vi "Teleop.vi"(10 "Match Info":T1={"Autonomous Elapsed Seconds"=0.0, "TeleOp Elapsed Seconds"=0.0, "Disabled Elapsed Seconds"=0.0, "Visited Autonomous"=FALSE, "Visited TeleOp"=FALSE, "Visited Disabled"=FALSE, "Autonomous Settings"={"Autonomous Style"=enum."Independent", "VI Refnum"=refnum}}, 11 "Call Context":T2) -> ()   [LabVIEW 2017]
doc: "This VI is called for each TeleOp packet received from the DS where the robot is not disabled. It is often used to read from the joysticks and update I/O or to update setpoints for timed control loops. It should complete and return within 20 milliseconds or it may miss DS packets."
uses:
  <vilib>/Rock Robotics/WPI/DriverStation/WPI_DriverStationDerivedRobotMode.ctl
  <vilib>/Rock Robotics/WPI/DriverStation/WPI_DriverStationMatch Info.ctl
  <vilib>/Rock Robotics/WPI/Utilities/WPI_GetSetVariantRefNum.vi
  <vilib>/Rock Robotics/WPI/ThirdParty/Phoenix-LabVIEW/Motor Controller/Get/CTRE_Phoenix_MotorController_GetVoltage.vi
  Robot Global Data.vi
  <vilib>/Rock Robotics/Network Tables/NT Write Boolean Array.vi
  <vilib>/Rock Robotics/Network Tables/NT Write Numeric Array.vi
  <vilib>/Rock Robotics/Network Tables/NT Read Boolean.vi
  <vilib>/Rock Robotics/Network Tables/NT Read Number.vi
  <vilib>/Rock Robotics/WPI/ThirdParty/Phoenix-LabVIEW/Motor Controller/Get/CTRE_Phoenix_MotorController_GetQuadratureData.vi
panel:
  out "Motor Out (x)":dbl
  in  "Input":bool
  out "Rotation":dbl
  out "Quadrature Position":i32
  out "Quadrature Velocity":i32
  out "Sample Slider 0":dbl(slide) scale=0.0..5.0
  out "Sample Boolean 1":bool
  out "Sample Boolean 0":bool
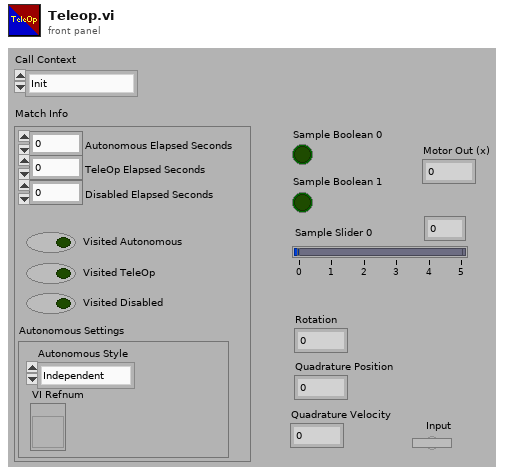
[diagram p1: front panel]
types:
  T1 = typedef "WPI_DriverStationMatch Info.ctl" = cluster{"Autonomous Elapsed Seconds":dbl, "TeleOp Elapsed Seconds":dbl, "Disabled Elapsed Seconds":dbl, "Visited Autonomous":bool, "Visited TeleOp":bool, "Visited Disabled":bool, "Autonomous Settings":cluster{"Autonomous Style":enum16{"Iterative", "Independent"}, "VI Refnum":refnum<vi>}}
  T2 = typedef "WPI_DriverStationDerivedRobotMode.ctl" = enum16{"Init", "Execute", "Stop"}
  T3 = typedef "WPI_RobotDriveDevRef.ctl" = cluster{"DevStatus":errorcluster, "Motors[]":T4[], "Square Inputs":bool, "Max Output":dbl}
  T4 = typedef "WPI_MotorControlDeviceRef.ctl" = cluster{"DeviceStatus":errorcluster, "Type":T5, "PWM":cluster{"PWM Channel":T6, "DeadBand":T7}, "CAN":cluster{"Device Number":u8, "SetOutput VI Ref":variant, "GetOutput VI Ref":variant, "Enable VI Ref":variant, "Disable VI Ref":variant, "Data":variant}, "Invert":bool, "DIO PWM":cluster{"PWM \"Enable\" Channel":T6, "DIOChannel":T8, "PWM Rate":dbl}}
  T5 = typedef "WPI_MotorControlType.ctl" = enum16{"PWM", "CAN", "DIO PWM"}
  T6 = typedef "FPGA_DIOPWMChannel.ctl" = enum8{"PWM 0", "PWM 1", "PWM 2", "PWM 3", "PWM 4", "PWM 5", "PWM 6", "PWM 7", "PWM 8", "PWM 9", "PWM MXP 0", "PWM MXP 1", "PWM MXP 2", "PWM MXP 3", "PWM MXP 4", "PWM MXP 5", "PWM MXP 6", "PWM MXP 7", "PWM MXP 8", "PWM MXP 9", "Invalid"}
  T7 = typedef "WPI_PWMDeadband.ctl" = cluster{"Name":string, "maxPositivePwm":i32, "minPositivePwm":i32, "centerPwm":i32, "maxNegativePwm":i32, "minNegativePwm":i32, "angularRange":u16}
  T8 = typedef "FPGA_DIOChannel.ctl" = enum8{"DIO 0", "DIO 1", "DIO 2", "DIO 3", "DIO 4", "DIO 5", "DIO 6", "DIO 7", "DIO 8", "DIO 9", "DIO MXP 0", "DIO MXP 1", "DIO MXP 2", "DIO MXP 3", "DIO MXP 4", "DIO MXP 5", "DIO MXP 6", "DIO MXP 7", "DIO MXP 8", "DIO MXP 9", "DIO MXP 10", "DIO MXP 11", "DIO MXP 12", "DIO MXP 13", "DIO MXP 14", "DIO MXP 15", "SPI Port CS1", "SPI Port CS2", "SPI Port CS3", "SPI Port MISO", "SPI Port MOSI", "Invalid"}
  T9 = typedef "WPI_JoystickDevRef.ctl" = cluster{"Device":T10}
  T10 = typedef "WPI_JoystickDeviceEnum.ctl" = enum16{"USB 0", "USB 1", "USB 2", "USB 3", "USB 4", "USB 5"}
  T11 = cluster{"Buttons[0]":bool, "Buttons[1]":bool, "Buttons[2]":bool, "Buttons[3]":bool, "Buttons[4]":bool, "Buttons[5]":bool, "Buttons[6]":bool, "Buttons[7]":bool, "Buttons[8]":bool}
  T12 = cluster{"Percent Output":dbl, "Output Voltage":dbl, "Bus Voltage":dbl}
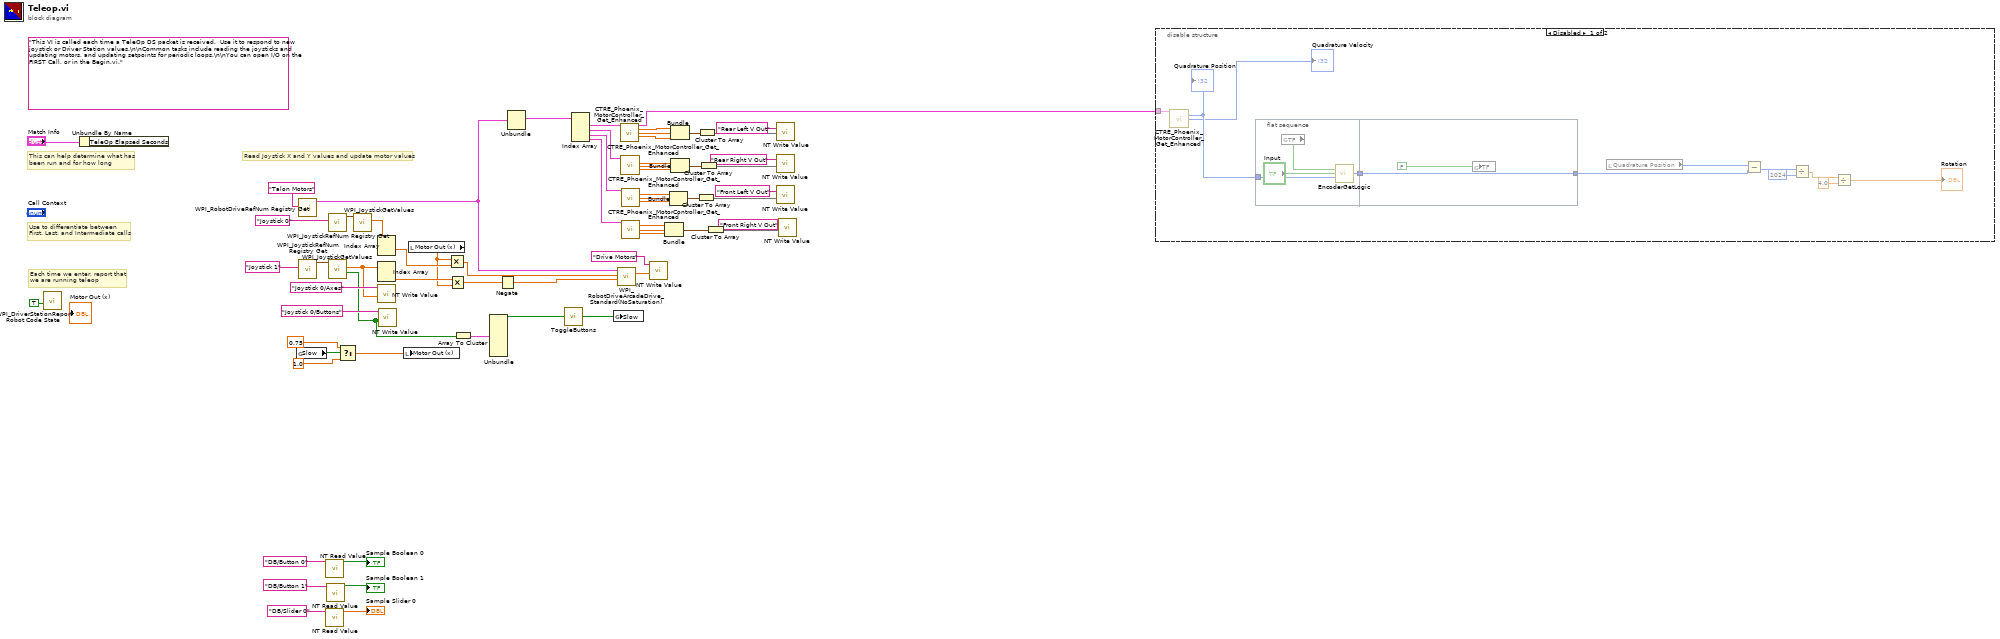
[diagram p0: block diagram]
diagram:
  (unwired) "This VI is called each time a TeleOp DS packet is received.  Use it to respond to new joystick or Driver Station values.\n\nCommon tasks include reading the joysticks and updating motors, and updating setpoints for periodic loops.\n\nYou can open I/O on the FIRST Call, or in the Begin.vi."
  # "Each time we enter, report that\nwe are running teleop"
  # "Use to differentiate between\nFirst, Last, and Intermediate calls"
  # "This can help determine what has\nbeen run and for how long"
  # "Read Joystick X and Y values and update motor values"
  n1 = call <vilib>:"WPI_DriverStationReport Robot Code State.vi"("TeleOp"=TRUE ("Autonomous")) -> ()  [unwired: 10 in, 1 out]
  n2 = Unbundle By Name("Match Info") -> ()  [unwired: 1 out]
  n3 = global read "Robot Global Data.vi" "Slow"() -> (w10:bool)
  n4 = call <vilib>:"WPI_RobotDriveRefNum Registry Get.vi"("refnum name"="Talon Motors") -> ("RobotDriveDevRef"=w46:T3)  [unwired: 1 in, 9 out]
  n5 = call <vilib>:"WPI_JoystickRefNum Registry Get.vi"("refnum name"="Joystick 1") -> ("JoystickDevRef"=w61:T9)  [unwired: 1 in, 9 out]
  n6 = call-poly <vilib>:"NT Read Value.vi"("Name"="DB/Button 0" ("refnum name")) -> ("Boolean"=→"Sample Boolean 0":bool)  [unwired: 9 in, 1 out]
  n7 = call-poly <vilib>:"NT Read Value.vi"("Name"="DB/Slider 0" ("refnum name")) -> ("Numeric"=→"Sample Slider 0":dbl)  [unwired: 9 in, 1 out]
  n8 = call-poly <vilib>:"NT Read Value.vi"("Name"="DB/Button 1" ("refnum name")) -> ("Boolean"=→"Sample Boolean 1":bool)  [unwired: 9 in, 1 out]
  n9 = call <vilib>:"WPI_JoystickGetValues.vi"("JoystickDevRef"=w61) -> ("Buttons"=w48:bool[], "Axes"=w57:dbl[])  [unwired: 6 in, 3 out]
  n10 = call <vilib>:"WPI_JoystickRefNum Registry Get.vi"("refnum name"="Joystick 0") -> ("JoystickDevRef"=w43:T9)  [unwired: 9 in, 1 out]
  n11 = Select(t=0.75, s=w10, f=1.0) -> (s? t:f=w7:dbl)
  n12 = call <vilib>:"WPI_JoystickGetValues.vi"("JoystickDevRef"=w43) -> ("Axes"=w42:dbl[])  [unwired: 6 in, 4 out]
  n13 = Index Array(array=w42) -> (element #1=w5:dbl)  [unwired: 2 in, 1 out]
  n14 = Index Array(array=w57) -> (element #2=w4:dbl)  [unwired: 2 in, 1 out]
  n15 = call-poly <vilib>:"NT Write Value.vi"("Numeric Array"=w57, "Name"="Joystick 0/Axes") -> ()  [unwired: 9 in, 1 out]
  n16 = call-poly <vilib>:"NT Write Value.vi"("Boolean Array"=w48, "Name"="Joystick 0/Buttons") -> ()  [unwired: 9 in, 1 out]
  n17 = local write "Motor Out (x)"(w7) -> ()
  n18 = local read "Motor Out (x)"() -> (w3:dbl)
  n19 = Multiply(x=w3, y=w5) -> (x*y=w6:dbl)
  n20 = Multiply(x=w4, y=w3) -> (x*y=w2:dbl)
  n21 = Array To Cluster(array=w48) -> (cluster=w47:T11)
  n22 = Unbundle(w47) -> ("Buttons[0]"=w12:bool)  [unwired: 8 out]
  n23 = Negate(x=w2) -> (-x=w1:dbl)
  n24 = Unbundle(w46) -> ("Motors[]"=w45:T4[])  [unwired: 3 out]
  n25 = call <vilib>:"ToggleButtons.vi"("Input 1"=w12) -> ("Output 1"=w11:bool)
  n26 = Index Array(array=w45) -> (element #1=w44:T4, element #2=w40:T4, element #3=w39:T4, element #4=w38:T4)  [unwired: 4 in]
  n27 = global write "Robot Global Data.vi" "Slow"(w11) -> ()
  n28 = call <vilib>:"WPI_RobotDriveArcadeDrive_Standard(NoSaturation).vi"("Y axis value"=w1, "X axis value"=w6, "RobotDriveDevRef"=w46) -> ("Motor Values"=w50:dbl[])  [unwired: 1 in, 7 out]
  n29 = call-poly <vilib>:"CTRE_Phoenix_MotorController_Get_Enhanced.vi"("PhoenixMotorControlDevRef"=w44) -> ("PhoenixMotorControlDevRef"=w13:T4, "Percent Output"=w18:dbl, "Output Voltage"=w17:dbl, "Bus Voltage"=w16:dbl)  [unwired: 10 in, 1 out]
  n30 = call-poly <vilib>:"CTRE_Phoenix_MotorController_Get_Enhanced.vi"("PhoenixMotorControlDevRef"=w40) -> ("Percent Output"=w22:dbl, "Output Voltage"=w23:dbl, "Bus Voltage"=w21:dbl)  [unwired: 10 in, 2 out]
  n31 = call-poly <vilib>:"CTRE_Phoenix_MotorController_Get_Enhanced.vi"("PhoenixMotorControlDevRef"=w39) -> ("Percent Output"=w28:dbl, "Output Voltage"=w27:dbl, "Bus Voltage"=w26:dbl)  [unwired: 10 in, 2 out]
  n32 = call-poly <vilib>:"CTRE_Phoenix_MotorController_Get_Enhanced.vi"("PhoenixMotorControlDevRef"=w38) -> ("Percent Output"=w33:dbl, "Output Voltage"=w32:dbl, "Bus Voltage"=w31:dbl)  [unwired: 10 in, 2 out]
  n33 = call-poly <vilib>:"NT Write Value.vi"("Numeric Array"=w50, "Name"="Drive Motors") -> ()  [unwired: 9 in, 1 out]
  n34 = Bundle("Percent Output"=w33, "Output Voltage"=w32, "Bus Voltage"=w31) -> (w30:T12)  [unwired: 1 in]
  n35 = Bundle("Percent Output"=w28, "Output Voltage"=w27, "Bus Voltage"=w26) -> (w25:T12)  [unwired: 1 in]
  n36 = Bundle("Percent Output"=w18, "Output Voltage"=w17, "Bus Voltage"=w16) -> (w15:T12)  [unwired: 1 in]
  n37 = Bundle("Percent Output"=w22, "Output Voltage"=w23, "Bus Voltage"=w21) -> (w20:T12)  [unwired: 1 in]
  n38 = Cluster To Array(cluster=w25) -> (array=w24:dbl[])
  n39 = Cluster To Array(cluster=w15) -> (array=w14:dbl[])
  n40 = Cluster To Array(cluster=w20) -> (array=w19:dbl[])
  n41 = Cluster To Array(cluster=w30) -> (array=w29:dbl[])
  n42 = call-poly <vilib>:"NT Write Value.vi"("Numeric Array"=w19, "Name"="Rear Right V Out") -> ()  [unwired: 9 in, 1 out]
  n43 = call-poly <vilib>:"NT Write Value.vi"("Numeric Array"=w24, "Name"="Front Left V Out") -> ()  [unwired: 9 in, 1 out]
  n44 = call-poly <vilib>:"NT Write Value.vi"("Numeric Array"=w14, "Name"="Rear Left V Out") -> ()  [unwired: 9 in, 1 out]
  n45 = call-poly <vilib>:"NT Write Value.vi"("Numeric Array"=w29, "Name"="Front Right V Out") -> ()  [unwired: 9 in, 1 out]
  n46 = disable-structure shown="Disabled" {
    disable-tunnel: w13 -> [w65 _]
    frame Disabled {
      n47 = call-poly <vilib>:"CTRE_Phoenix_MotorController_Get_Enhanced.vi"("PhoenixMotorControlDevRef"=w65) -> ("Quadrature Position"=w67:i32, "Quadrature Velocity"=→"Quadrature Velocity":i32)  [unwired: 11 in, 2 out]
      "Quadrature Position" <- w67
      n48 = flat-sequence {
        tunnel: w67 -> [w79]
        tunnel: [w78] -> w75
        tunnel: [w81] -> w68
        tunnel: w75 -> [w81]
        frame #0 {
          n49 = global read "Robot Global Data.vi" "TF"() -> (w76:bool)
          n50 = call <vilib>:"EncoderGetLogic.vi"("Global Variable"=w76, "Sensor Input"="Input", "Quad Position"=w79) -> ("Variable of Comparison"=w78:i32)  [unwired: 12 in]
        }
        frame #1 {
          n51 = global write "Robot Global Data.vi" "TF"(FALSE) -> ()
        }
      }
      n52 = local read "Quadrature Position"() -> (w74:i32)
      n53 = Subtract(x=w74, y=w68) -> (x-y=w73:i32)
      n54 = Divide(x=w73, y=1024) -> (x/y=w71:dbl)
      n55 = Divide(x=w71, y=4.0) -> (x/y=→"Rotation":dbl)
    }
    frame Enabled {
    }
  }
